vi "LinSpace.vi"(9 "Num Steps":i32, 10 "Max":dbl, 11 "Min":dbl) -> (3 "Array":dbl[](array[numeric]))   [LabVIEW 2012]
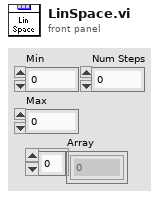
[diagram p1: front panel]
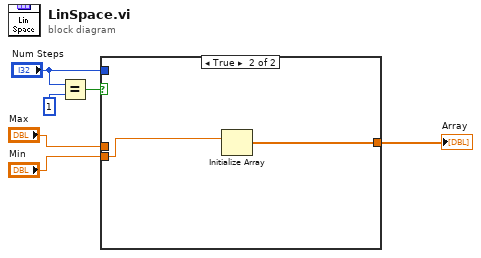
[diagram p0: block diagram]
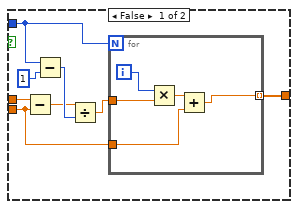
[diagram p2: hidden frame]
diagram:
  n1 = Equal?(x="Num Steps", y=1) -> (x = y?=w5:bool)
  n2 = case shown="True" w5 {
    tunnel: "Num Steps" -> [w12 _]
    tunnel: "Max" -> [w14 _]
    tunnel: "Min" -> [w8 w21]
    tunnel: [w7 w20] -> w1
    frame False {
      n3 = Subtract(x=w14, y=w8) -> (x-y=w10:dbl)
      n4 = Subtract(x=w12, y=1) -> (x-y=w11:i32)
      n5 = Divide(x=w10, y=w11) -> (x/y=w9:dbl)
      n6 = for {
        N: w12 -> [_]
        tunnel: w9 -> [w19]
        tunnel: w8 -> [w16]
        tunnel: [w15] -> w7 mode=indexing
        i -> [w18]
        n7 = Multiply(x=w18, y=w19) -> (x*y=w17:dbl)
        n8 = Add(x=w17, y=w16) -> (x+y=w15:dbl)
      }
    }
    frame True {
      n9 = Initialize Array(w21) -> (w20:dbl[])  [unwired: 1 in]
    }
  }
  "Array" <- w1
